vi "test_CRIO daqmx PWM Open Collector.vi"(8 "Error In":errorcluster) -> (0 "Error Out":errorcluster)   [LabVIEW 2023]
uses:
  Series/Series Base/Series Base.lvclass
  DIO/Virtual DIO/Virt PWM Fixed Freq Generator/Virt DAQmx Fixed Freq PWM Generator.lvclass
  DIO/DO DAQmx Fixed Freq PWM CFG/DO DAQmx Fixed Freq PWM CFG.lvclass
  Sample Tasks/Sample PWM Fan/Sample PWM Fan.lvclass
  Series/Series Base/Series Base.lvclass/Series Base.ctl
  Task/Task Base/Task Base.lvclass/Task Base.ctl
  <vilib>/Utility/error.llb/Error Cluster From Error Code.vi
  Task/Task Base/Task Base.lvclass
  Measure and Stimulus Subsystems/Measure and Stimulus Subsystems.lvclass
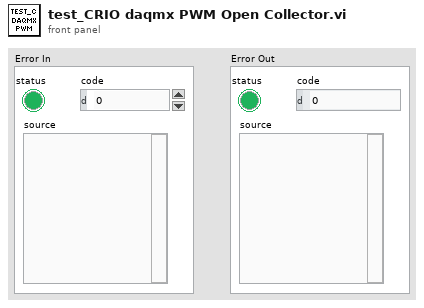
[diagram p1: front panel]
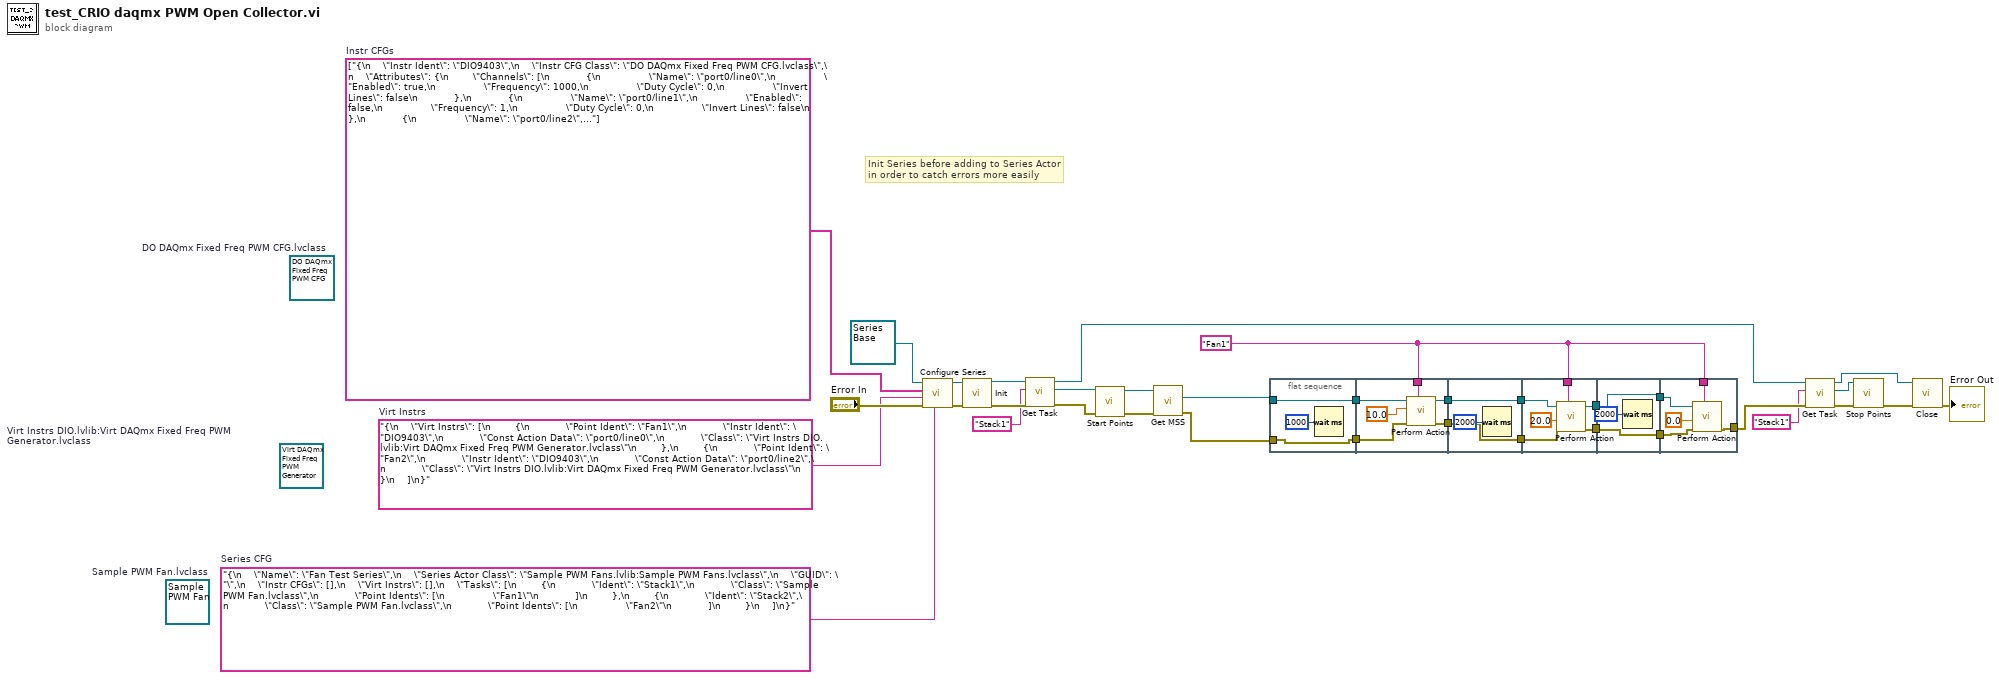
[diagram p0: block diagram]
diagram:
  (unwired) refnum<class "Sample PWM Fan.lvclass"> refnum  # Sample PWM Fan.lvclass
  w12 = "Fan1" ("Point Ident")
  (unwired) refnum<class "DO DAQmx Fixed Freq PWM CFG.lvclass"> refnum  # DO DAQmx Fixed Freq PWM CFG.lvclass
  (unwired) refnum<class "Virt DAQmx Fixed Freq PWM Generator.lvclass"> refnum  # Virt Instrs DIO.lvlib:Virt DAQmx Fixed Freq PWM Generator.lvclass
  w31 = "{\n    \"Virt Instrs\": [\n        {\n            \"Point Ident\": \"Fan1\",\n            \"Instr Ident\": \"DIO9403\",\n            \"Const Action Data\": \"port0/line0\",\n            \"Class\": \"Virt Instrs DIO.lvlib:Virt DAQmx Fixed Freq PWM Generator.lvclass\"\n        },\n        {\n            \"Point Ident\": \"Fan2\",\n            \"Instr Ident\": \"DIO9403\",\n            \"Const Action Data\": \"port0/line2\",\n            \"Class\": \"Virt Instrs DIO.lvlib:Virt DAQmx Fixed Freq PWM Generator.lvclass\"\n        }\n    ]\n}"  # Virt Instrs
  w30 = string[] ["{\n    \"Instr Ident\": \"DIO9403\",\n    \"Instr CFG Class\": \"DO DAQmx Fixed Freq PWM CFG.lvclass\",\n    \"Attributes\": {\n        \"Channels\": [\n            {\n                \"Name\": \"port0/line0\",\n                \"Enabled\": true,\n                \"Frequency\": 1000,\n                \"Duty Cycle\": 0,\n                \"Invert Lines\": false\n            },\n            {\n                \"Name\": \"port0/line1\",\n                \"Enabled\": false,\n                \"Frequency\": 1,\n                \"Duty Cycle\": 0,\n                \"Invert Lines\": false\n            },\n            {\n                \"Name\": \"port0/line2\",\n                \"Enabled\": true,\n                \"Frequency\": 600,\n                \"Duty Cycle\": 0,\n                \"Invert Lines\": false\n            }\n        ],\n        \"Timing\": {\n            \"Mode\": \"Sample Clock\",\n            \"Samples per Channel\": 10000,\n            \"Sample Mode\": \"Continuous Samples\",\n            \"Sample Rate\": 100000,\n            \"Sample Clock Source\": \"OnboardClock\",\n            \"Active Edge\": \"Rising\"\n        },\n        \"Trigger\": {\n            \"Trigger Type\": \"No Trigger\"\n        },\n        \"Generation\": {\n            \"Regen Mode\": \"Allow Regeneration\"\n        }\n    }\n}"]  # Instr CFGs
  w29 = "{\n    \"Name\": \"Fan Test Series\",\n    \"Series Actor Class\": \"Sample PWM Fans.lvlib:Sample PWM Fans.lvclass\",\n    \"GUID\": \"\",\n    \"Instr CFGs\": [],\n    \"Virt Instrs\": [],\n    \"Tasks\": [\n        {\n            \"Ident\": \"Stack1\",\n            \"Class\": \"Sample PWM Fan.lvclass\",\n            \"Point Idents\": [\n                \"Fan1\"\n            ]\n        },\n        {\n            \"Ident\": \"Stack2\",\n            \"Class\": \"Sample PWM Fan.lvclass\",\n            \"Point Idents\": [\n                \"Fan2\"\n            ]\n        }\n    ]\n}"  # Series CFG
  # "Init Series before adding to Series Actor\nin order to catch errors more easily"
  n1 = call "Configure Series.vi"("Series CFG"=w29, "error in (no error)"="Error In", "Virt Instrs CFG"=w31, "Instr CFGs"=w30, "HAL GOOP4:Series Base in"=refnum<class "Series Base.lvclass"> refnum ("HAL GOOP4.lvlib:Study Base.lvclass")) -> ("error out"=w34:errorcluster, "HAL GOOP4:Series Base out"=w32:refnum<class "Series Base.lvclass">)  [unwired: 5 in]
  n2 = call-dynamic "Init.vi"("error in"=w34, "HAL GOOP4:Series Base in"=w32) -> ("error out"=w27:errorcluster, "HAL GOOP4:Series Base out"=w14:refnum<class "Series Base.lvclass">)  [unwired: 8 in]
  n3 = call "Get Task.vi"("error in (no error)"=w27, "Task Name"="Stack1" ("key"), "Series Base in"=w14) -> ("error out"=w10:errorcluster, "Task"=w11:refnum<class "Task Base.lvclass">, "Series Base out"=w5:refnum<class "Series Base.lvclass">)  [unwired: 6 in]
  n4 = call-dynamic "Start Points.vi"("error in"=w10, "Task Base in"=w11) -> ("error out"=w9:errorcluster, "Task Base out"=w7:refnum<class "Task Base.lvclass">)  [unwired: 8 in]
  n5 = call "Get MSS.vi"("error in (no error)"=w9, "Task Base in"=w7) -> ("error out"=w13:errorcluster, "MSS"=w8:refnum<class "Measure and Stimulus Subsystems.lvclass">)  [unwired: 7 in, 1 out]
  n6 = flat-sequence {
    tunnel: w8 -> [w38]
    tunnel: [w38] -> w26
    tunnel: w13 -> [w36]
    tunnel: [w36] -> w25
    tunnel: w26 -> [w44]
    tunnel: w25 -> [w42]
    tunnel: [w41] -> w23
    tunnel: [w40] -> w21
    tunnel: w12 -> [w39]
    tunnel: [w46] -> w24
    tunnel: w23 -> [w46]
    tunnel: [w45] -> w22
    tunnel: w21 -> [w45]
    tunnel: w24 -> [w52]
    tunnel: w22 -> [w51]
    tunnel: [w50] -> w20
    tunnel: [w49] -> w19
    tunnel: w12 -> [w48]
    tunnel: w20 -> [w55]
    tunnel: w19 -> [w54]
    tunnel: [w55] -> w18
    tunnel: [w54] -> w17
    tunnel: w18 -> [w60]
    tunnel: w17 -> [w59]
    tunnel: [w58] -> w16
    tunnel: w12 -> [w57]
    frame #0 {
      n7 = Wait (ms)(milliseconds to wait=u32 1000) -> ()  [unwired: 1 out]
    }
    frame #1 {
      n8 = call "Perform Action.vi"("Point Ident"=w39, "error in"=w42, "Input"=10.0, "MSS in"=w44) -> ("error out"=w40:errorcluster, "MSS out"=w41:refnum<class "Measure and Stimulus Subsystems.lvclass">)  [unwired: 5 in, 1 out]
    }
    frame #2 {
      n9 = Wait (ms)(milliseconds to wait=u32 2000) -> ()  [unwired: 1 out]
    }
    frame #3 {
      n10 = call "Perform Action.vi"("Point Ident"=w48, "error in"=w51, "Input"=20.0, "MSS in"=w52) -> ("error out"=w49:errorcluster, "MSS out"=w50:refnum<class "Measure and Stimulus Subsystems.lvclass">)  [unwired: 5 in, 1 out]
    }
    frame #4 {
      n11 = Wait (ms)(milliseconds to wait=u32 2000) -> ()  [unwired: 1 out]
    }
    frame #5 {
      n12 = call "Perform Action.vi"("Point Ident"=w57, "error in"=w59, "Input"=0.0, "MSS in"=w60) -> ("error out"=w58:errorcluster)  [unwired: 5 in, 2 out]
    }
  }
  n13 = call "Get Task.vi"("error in (no error)"=w16, "Task Name"="Stack1" ("key"), "Series Base in"=w5) -> ("error out"=w6:errorcluster, "Task"=w2:refnum<class "Task Base.lvclass">, "Series Base out"=w1:refnum<class "Series Base.lvclass">)  [unwired: 6 in]
  n14 = call-dynamic "Stop Points.vi"("error in"=w6, "Task Base in"=w2) -> ("error out"=w3:errorcluster)  [unwired: 8 in, 1 out]
  n15 = call-dynamic "Close.vi"("error in"=w3, "Series Base in"=w1) -> ("error out"=→"Error Out":errorcluster)  [unwired: 8 in, 1 out]
